vi "time_scan_init.vi"(8 "timesteps":dbl[](array[numeric]), 9 "stage_t0_position":dbl, 10 "current scan idx":i32, 11 "current step idx":i32) -> (0 "current time step":dbl, 1 "current time step position on stage":dbl, 2 "current scan idx out":u16, 3 "current step idx out":u16)   [LabVIEW 2018]
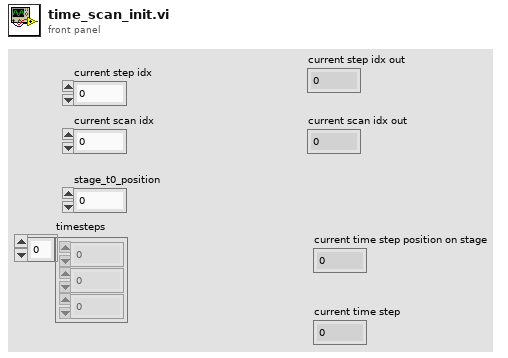
[diagram p1: front panel]
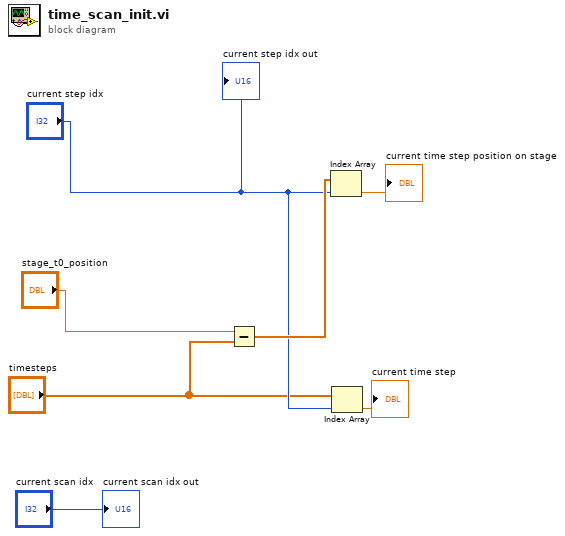
[diagram p0: block diagram]
diagram:
  n1 = Subtract(x="stage_t0_position", y="timesteps") -> (x-y=w6:dbl[])
  n2 = Index Array(array=w6, index="current step idx") -> (element=→"current time step position on stage":dbl)
  n3 = Index Array(array="timesteps", index="current step idx") -> (element=→"current time step":dbl)
  "current step idx out" <- "current step idx"
  "current scan idx out" <- "current scan idx"
